vi "SDKSID4_UtilsSDK_ErrorManager.vi"(1 "error IN":errorcluster caption="Error IN", 2 "VI PathFile":path, 3 "ErrorCode":i32) -> (0 "error OUT":errorcluster caption="Error OUT")   [LabVIEW 2013]
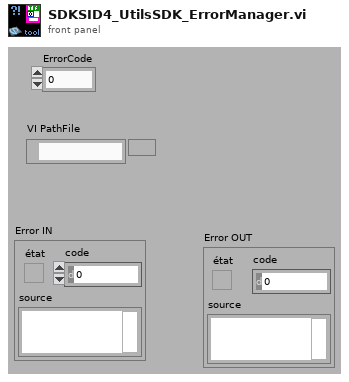
[diagram p1: front panel]
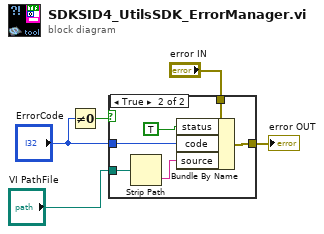
[diagram p0: block diagram]
diagram:
  n1 = Not Equal To 0?(x="ErrorCode") -> (x != 0?=w5:bool)
  n2 = case shown="True" w5 {
    tunnel: "error IN" -> [w6 w12]
    tunnel: "ErrorCode" -> [_ w11]
    tunnel: [w6 w8] -> w2
    tunnel: "VI PathFile" -> [_ w7]
    frame False {
    }
    frame True {
      n3 = Strip Path(path=w7) -> (name=w9:string)  [unwired: 1 out]
      n4 = Bundle By Name(cluster=w12, "status"=TRUE, "code"=w11, "source"=w9) -> (w8:errorcluster)
    }
  }
  "error OUT" <- w2
